vi "Create ipf File.vi"(2 "error in":errorcluster, 3 "Default ipf file path":path) -> (0 "error out":errorcluster, 1 "ipf file path":path)   [LabVIEW 2018]
doc: "This creats IPF file in selected location"
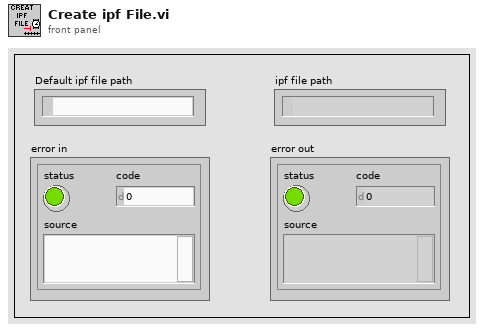
[diagram p1: front panel]
types:
  T1 = enum32{"invalid app kind", "Development System", "Run Time System", "Student Edition", "Embedded LabVIEW", "Evaluation", "Custom"}
  T2 = enum16{"open", "replace", "create", "open or create", "replace or create", "replace or create with confirmation"}
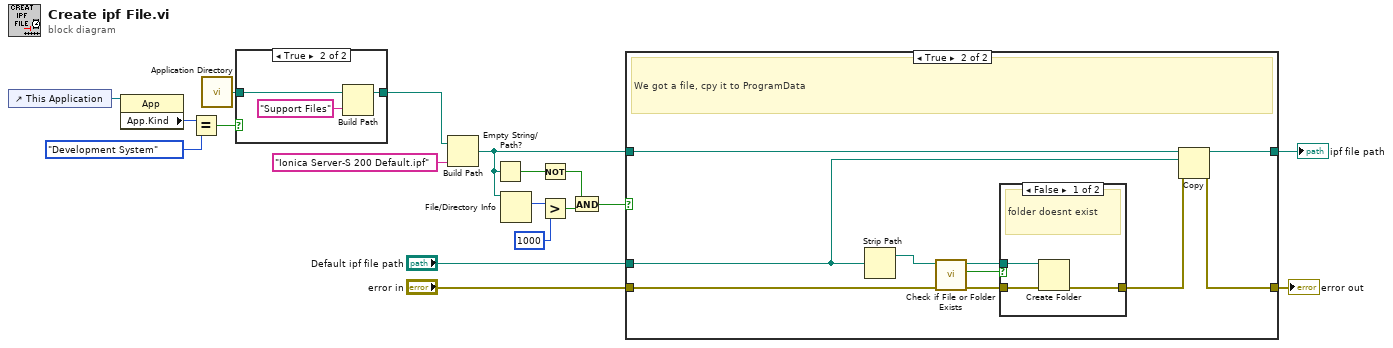
[diagram p0: block diagram]
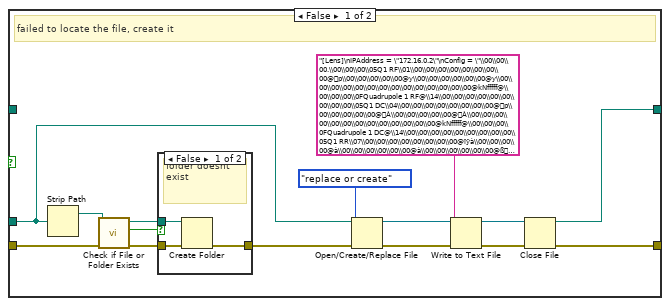
[diagram p3: hidden frame]
diagram:
  n1 = control-ref of="This Application"() -> (w6:refnum<vi>)
  n2 = property class="App"(reference=w6) -> ("App.Kind"=w5:T1)  [unwired: 1 in, 2 out]
  n3 = Equal?(x=w5, y=T1."Development System" ("Application:Kind")) -> (x = y?=w3:bool)
  n4 = call <vilib>:"Application Directory.vi"() -> ("Application Directory"=w2:path)
  n5 = case shown="True" w3 {
    tunnel: w2 -> [w19 w22]
    tunnel: [w19 w21] -> w1
    frame False {
    }
    frame True {
      n6 = Build Path(base path=w22, name or relative path="Support Files") -> (appended path=w21:path)
    }
  }
  n7 = Build Path(base path=w1, name or relative path="Ionica Server-S 200 Default.ipf") -> (appended path=w12:path)
  n8 = Empty String/Path?(string/path=w12) -> (empty?=w17:bool)
  n9 = File/Directory Info(path=w12) -> (size=w15:i64)  [unwired: 1 in, 6 out]
  n10 = Not(x=w17) -> (.not. x?=w16:bool)
  n11 = Greater?(x=w15, y=i64 1000) -> (0:w18:bool)
  n12 = And(x=w16, y=w18) -> (x .and. y?=w7:bool)
  n13 = case shown="True" w7 {
    tunnel: w12 -> [_ w51]
    tunnel: "error in" -> [w25 w47]
    tunnel: [w33 w50] -> w10
    tunnel: [w31 w49] -> w9
    tunnel: "Default ipf file path" -> [w24 w42]
    frame False {
      # "failed to locate the file, create it"
      n14 = Strip Path(path=w24) -> (stripped path=w28:path)  [unwired: 1 out]
      n15 = call <vilib>:"Check if File or Folder Exists.vi"("error in (no error)"=w25, "path"=w28) -> ("error out"=w30:errorcluster, "file or folder exists?"=w29:bool, "dup path"=w27:path)  [unwired: 7 in]
      n16 = case shown="False" w29 {
        tunnel: [w40 w41] -> w26
        tunnel: w30 -> [w39 w41]
        tunnel: w27 -> [w38 _]
        frame False {
          # "folder doesnt exist"
          n17 = Create Folder(path (use dialog)=w38, error in=w39) -> (error out=w40:errorcluster)  [unwired: 1 in, 2 out]
        }
        frame True {
        }
      }
      n18 = Open/Create/Replace File(file path (use dialog)=w24, error in=w26, operation (0:open)=T2."replace or create") -> (refnum out=w35:refnum<file>, error out=w36:errorcluster)  [unwired: 3 in, 1 out]
      n19 = Write to Text File(file (use dialog)=w35, text="[Lens]\nIPAddress = \"172.16.0.2\"\nConfig = \"\\00\\00\\00.\\00\\00\\00\\05Q1 RF\\01\\00\\00\\00\\00\\00\\00\\00\\00@p\\00\\00\\00\\00\\00@y\\00\\00\\00\\00\\00\\00@y\\00\\00\\00\\00\\00\\00\\00\\00\\00\\00\\00\\00\\00\\00@kNfffff@\\00\\00\\00\\0FQuadrupole 1 RF@\\14\\00\\00\\00\\00\\00\\00\\00\\00\\00\\05Q1 DC\\04\\00\\00\\00\\00\\00\\00\\00\\00@p\\00\\00\\00\\00\\00@À\\00\\00\\00\\00\\00@À\\00\\00\\00\\00\\00\\00\\00\\00\\00\\00\\00\\00\\00@kNfffff@\\00\\00\\00\\0FQuadrupole 1 DC@\\14\\00\\00\\00\\00\\00\\00\\00\\00\\00\\05Q1 RR\\07\\00\\00\\00\\00\\00\\00\\00\\00@ïÿà\\00\\00\\00\\00@à\\00\\00\\00\\00\\00\\00@à\\00\\00\\00\\00\\00\\00@ßÀ\\00\\00\\00\\00?ð\\00\\00\\00\\00\\00\\00@\\00\\00\\00\\0FQuadrupole 1 PW@\\14\\00\\00\\00\\00\\00\\00\\00\\00\\00\\05Q2 RF\\02\\00\\00\\00\\00\\00\\00\\00\\00@p\\00\\00\\00\\00\\00@y\\00\\00\\00\\00\\00\\00@y\\00\\00\\00\\00\\00\\00\\00\\00\\00\\00\\00\\00\\00\\00@kNfffff@\\00\\00\\00\\0FQuadrupole 2 RF@\\14\\00\\00\\00\\00\\00\\00\\00\\00\\00\\05Q2 DC\\05\\00\\00\\00\\00\\00\\00\\00\\00@p\\00\\00\\00\\00\\00@À\\00\\00\\00\\00\\00@À\\00\\00\\00\\00\\00\\00\\00\\00\\00\\00\\00\\00\\00@kNfffff@\\00\\00\\00\\0FQuadrupole 2 DC@\\14\\00\\00\\00\\00\\00\\00\\00\\00\\00\\05Q2 RR\t\\00\\00\\00\\00\\00\\00\\00\\00@ïÿà\\00\\00\\00\\00@à\\00\\00\\00\\00\\00\\00@à\\00\\00\\00\\00\\00\\00@ß¹À\\00\\00\\00\\00?ð\\00\\00\\00\\00\\00\\00@\\00\\00\\00\\0FQuadrupole 2 PW@\\14\\00\\00\\00\\00\\00\\00\\00\\00\\00\\05M1 RF\\03\\00\\00\\00\\00\\00\\00\\00\\00@@\\00\\00\\00\\00\\00@Y\\00\\00\\00\\00\\00\\00@Y\\00\\00\\00\\00\\00\\00\\00\\00\\00\\00\\00\\00\\00\\00@-ffffff\\06\\00\\00\\00\\0EMultipole 1 RF@\\14\\00\\00\\00\\00\\00\\00\\00\\00\\00\\02EV\\14Ài\\00\\00\\00\\00\\00\\00@i\\00\\00\\00\\00\\00\\00\\00\\00\\00\\00\\00\\00\\00\\00\\00\\00\\00\\00\\00\\00\\00\\00@à\\00\\00\\00\\00\\00\\00ÀPlÌÌÌÌÍ\\07\\00\\00\\00\\10Entrance Voltage@\\14\\00\\00\\00\\00\\00\\00\\00\\00\\00\\02ED\\15Ày\\00\\00\\00\\00\\00\\00@y\\00\\00\\00\\00\\00\\00\\00\\00\\00\\00\\00\\00\\00\\00\\00\\00\\00\\00\\00\\00\\00\\00@à\\00\\00\\00\\00\\00\\00À``\\00\\00\\00\\00\\00\\07\\00\\00\\00\\0ANot Used 1@\\14\\00\\00\\00\\00\\00\\00\\00\\00\\00\\02M1\\13Ày\\00\\00\\00\\00\\00\\00@y\\00\\00\\00\\00\\00\\00\\00\\00\\00\\00\\00\\00\\00\\00\\00\\00\\00\\00\\00\\00\\00\\00@à\\00\\00\\00\\00\\00\\00ÀPfffffg\\07\\00\\00\\00\\0BMultipole 1@\\14\\00\\00\\00\\00\\00\\00\\00\\00\\00\\02L1\\12Ày\\00\\00\\00\\00\\00\\00@y\\00\\00\\00\\00\\00\\00\\00\\00\\00\\00\\00\\00\\00\\00\\00\\00\\00\\00\\00\\00\\00\\00@ßþ\\00\\00\\00\\00\\00ÀPy\\07\\00\\00\\00\\10Multipole Lens 1@\\14\\00\\00\\00\\00\\00\\00\\00\\00\\00\\02M2\\16Ày\\00\\00\\00\\00\\00\\00@y\\00\\00\\00\\00\\00\\00\\00\\00\\00\\00\\00\\00\\00\\00\\00\\00\\00\\00\\00\\00\\00\\00@ß÷Êé\\13\\1AÀPjü-ÙÊ\\07\\00\\00\\00\\0BMultipole 2@\\14\\00\\00\\00\\00\\00\\00\\00\\00\\00\\02L2\\0BÀy\\00\\00\\00\\00\\00\\00@y\\00\\00\\00\\00\\00\\00\\00\\00\\00\\00\\00\\00\\00\\00\\00\\00\\00\\00\\00\\00\\00\\00@à\\00\\00\\00\\00\\00\\00ÀPzáG®\\14{\\07\\00\\00\\00\\10Multipole Lens 2@\\14\\00\\00\\00\\00\\00\\00\\00\\00\\00\\02PF\\0CÀy\\00\\00\\00\\00\\00\\00@y\\00\\00\\00\\00\\00\\00À0\\00\\00\\00\\00\\00\\00@0\\00\\00\\00\\00\\00\\00@à\\00\\00\\00\\00\\00\\01ÀPs33333\\07\\00\\00\\00\\0BPrefilter 1@\\14\\00\\00\\00\\00\\00\\00\\00\\00\\00\\02Q1\\06ÀbÀ\\00\\00\\00\\00\\00@bÀ\\00\\00\\00\\00\\00¿ð\\00\\00\\00\\00\\00\\00?ð\\00\\00\\00\\00\\00\\00@ßüÀ\\00\\00\\00\\00À`i\\0B\\00\\00\\00\\0CQuadrupole 1@\\14\\00\\00\\00\\00\\00\\00\\00\\00\\00\\05CC L1\\0DÀy\\00\\00\\00\\00\\00\\00@y\\00\\00\\00\\00\\00\\00\\00\\00\\00\\00\\00\\00\\00\\00\\00\\00\\00\\00\\00\\00\\00\\00@à\\00\\00\\00\\00\\00\\01ÀPs33333\\07\\00\\00\\00\\15Collision Cell Lens 1@\\14\\00\\00\\00\\00\\00\\00\\00\\00\\00\\05CC L2\\0EÀy\\00\\00\\00\\00\\00\\00@y\\00\\00\\00\\00\\00\\00ÀY\\00\\00\\00\\00\\00\\00@Y\\00\\00\\00\\00\\00\\00@à\\00\\00\\00\\00\\00\\01ÀPs33333\\07\\00\\00\\00\\15Collision Cell Lens 2@\\14\\00\\00\\00\\00\\00\\00\\00\\00\\00\\02CC\\17Ày\\00\\00\\00\\00\\00\\00@y\\00\\00\\00\\00\\00\\00ÀI\\00\\00\\00\\00\\00\\00@I\\00\\00\\00\\00\\00\\00@à\\04\\1B|S\\18ÀPmñLboÜ\\07\\00\\00\\00\\10Collision Energy@\\14\\00\\00\\00\\00\\00\\00\\00\\00\\00\\05CC AF\\0AÀy\\00\\00\\00\\00\\00\\00@y\\00\\00\\00\\00\\00\\00@I\\00\\00\\00\\00\\00\\00ÀI\\00\\00\\00\\00\\00\\00@à\\00\\00\\00\\00\\00\\01ÀPs33333\\07\\00\\00\\00\\0BAxial Field@\\14\\00\\00\\00\\00\\00\\00\\00\\00\\00\\05CC L3\\0FÀy\\00\\00\\00\\00\\00\\00@y\\00\\00\\00\\00\\00\\00ÀJ@\\00\\00\\00\\00\\00@J@\\00\\00\\00\\00\\00@ß÷Æ÷ýoÓÀPr\\10\\05 \\\\F\\07\\00\\00\\00\\15Collision Cell Lens 3@\\14\\00\\00\\00\\00\\00\\00\\00\\00\\00\\05CC L4\\10Ày\\00\\00\\00\\00\\00\\00@y\\00\\00\\00\\00\\00\\00ÀR \\00\\00\\00\\00\\00@R \\00\\00\\00\\00\\00@à\\00\\00\\00\\00\\00\\00ÀPlÌÌÌÌÍ\\07\\00\\00\\00\\15Collision Cell Lens 4@\\14\\00\\00\\00\\00\\00\\00\\00\\00\\00\\02Q2\\08ÀbÀ\\00\\00\\00\\00\\00@bÀ\\00\\00\\00\\00\\00ÀK\\00\\00\\00\\00\\00\\00@K\\00\\00\\00\\00\\00\\00@ßý\\00\\00\\00\\00\\00À`i\\0B\\00\\00\\00\\0CQuadrupole 2@\\14\\00\\00\\00\\00\\00\\00\\00\\00\\00\\02ID\\11Ày\\00\\00\\00\\00\\00\\00@y\\00\\00\\00\\00\\00\\00ÀY\\00\\00\\00\\00\\00\\00@Y\\00\\00\\00\\00\\00\\00@à\\00\\00\\00\\00\\00\\01ÀPs33333\\07\\00\\00\\00\\12Detector Deflector@\\14\\00\\00\\00\\00\\00\\00\\00\\00\\00\\04DISC @$\\00\\00\\00\\00\\00\\00@@\\00\\00\\00\\00\\00@4\\00\\00\\00\\00\\00\\00@4\\00\\00\\00\\00\\00\\00À\\14\\00\\00\\00\\00\\00\\00?ó®\\14záG®\\12\\00\\00\\00\\0DDiscriminator@$\\00\\00\\00\\00\\00\\00\\00\\00\\00\\02DV\"\\00\\00\\00\\00\\00\\00\\00\\00@«X\\00\\00\\00\\00\\00@¥\\18\\00\\00\\00\\00\\00@¥\\18\\00\\00\\00\\00\\00\\00\\00\\00\\00\\00\\00\\00\\00?Ú;HÂ\\05c´\\12\\00\\00\\00\\10Detector Voltage@$\\00\\00\\00\\00\\00\\00\\00\\00\\00\\08DET hornÈ\\00\\00\\00\\00\\00\\00\\00\\00@µ|\\00\\00\\00\\00\\00@µ|\\00\\00\\00\\00\\00@µ|\\00\\00\\00\\00\\00\\00\\00\\00\\00\\00\\00\\00\\00?Ú»)\\1EÏÇ0\\10\\00\\00\\00\\0DDetector Horn@$\\00\\00\\00\\00\\00\\00\\00\\00\\00\\06LS400A$\\00\\00\\00\\00\\00\\00\\00\\00@z@\\00\\00\\00\\00\\00@z@\\00\\00\\00\\00\\00@z@\\00\\00\\00\\00\\00\\00\\00\\00\\00\\00\\00\\00\\00@!\\04§Jy\\05@\\00\\00\\00\\18Lens Power Supply A +400@\\14\\00\\00\\00\\00\\00\\00\\00\\00\\00\\07LS-400A%Àz@\\00\\00\\00\\00\\00ÀT\\00\\00\\00\\00\\00\\00Àz@\\00\\00\\00\\00\\00Àz@\\00\\00\\00\\00\\00Àx%<SÆÀ!\\0Dö°ßk\\0E@\\00\\00\\00\\18Lens Power Supply A -400@\\14\\00\\00\\00\\00\\00\\00\\00\\00\\00\\06LS400B&\\00\\00\\00\\00\\00\\00\\00\\00@z@\\00\\00\\00\\00\\00@z@\\00\\00\\00\\00\\00@z@\\00\\00\\00\\00\\00\\00\\00\\00\\00\\00\\00\\00\\00@ ×Û%ö!@\\00\\00\\00\\18Lens Power Supply B +400@\\14\\00\\00\\00\\00\\00\\00\\00\\00\\00\\07LS-400B'Àz@\\00\\00\\00\\00\\00ÀT\\00\\00\\00\\00\\00\\00Àz@\\00\\00\\00\\00\\00Àz@\\00\\00\\00\\00\\00À´%\\03\\15$À ó©£xJ\\06@\\00\\00\\00\\19Lens Power Supply B  -400@\\14\\00\\00\\00\\00\\00\\00\\00\\00\\00\\06QPS800(\\00\\00\\00\\00\\00\\00\\00\\00@À\\00\\00\\00\\00\\00@À\\00\\00\\00\\00\\00@À\\00\\00\\00\\00\\00\\00\\00\\00\\00\\00\\00\\00\\00@\\11LÌÌÌÌÍ@\\00\\00\\00\\16Quad Power Supply +800@\\14\\00\\00\\00\\00\\00\\00\\00\\00\\00\\07QPS-800)ÀÀ\\00\\00\\00\\00\\00Àa\\00\\00\\00\\00\\00ÀÀ\\00\\00\\00\\00\\00ÀÀ\\00\\00\\00\\00\\00ÀÖ^ü^ýÀ\\11{ò\\19{ò\\1A@\\00\\00\\00\\16Quad Power Supply -800@\\14\\00\\00\\00\\00\\00\\00\\00\\00\\00\\02DG\\1A@D\\00\\00\\00\\00\\00\\00@rÀ\\00\\00\\00\\00\\00@T\\00\\00\\00\\00\\00\\00@T\\00\\00\\00\\00\\00\\00\\00\\00\\00\\00\\00\\00\\00\\00@@aë\\1E¸R \\00\\00\\00\\0ADrying Gas@@\\00\\00\\00\\00\\00\\00\\00\\00\\03NG1\\1B\\00\\00\\00\\00\\00\\00\\00\\00@@\\00\\00\\00\\00\\00\\00\\00\\00\\00\\00\\00\\00\\00\\00\\00\\00\\00\\00\\00\\00\\00\\00\\00\\00\\00\\00\\00\\00\\00@@aë\\1E¸R \\00\\00\\00\\0FNebulizer Gas 1@@\\00\\00\\00\\00\\00\\00\\00\\00\\03HG1\\1D\\00\\00\\00\\00\\00\\00\\00\\00@uà\\00\\00\\00\\00\\00\\00\\00\\00\\00\\00\\00\\00\\00\\00\\00\\00\\00\\00\\00\\00\\00\\00\\00\\00\\00\\00\\00\\00\\00@@aë\\1E¸R \\00\\00\\00\\0DHeating Gas 1@@\\00\\00\\00\\00\\00\\00\\00\\00\\03NG2\\1C\\00\\00\\00\\00\\00\\00\\00\\00@@\\00\\00\\00\\00\\00\\00\\00\\00\\00\\00\\00\\00\\00\\00\\00\\00\\00\\00\\00\\00\\00\\00\\00\\00\\00\\00\\00\\00\\00@@aë\\1E¸R \\00\\00\\00\\0FNebulizer Gas 2@@\\00\\00\\00\\00\\00\\00\\00\\00\\03HG2\\1E\\00\\00\\00\\00\\00\\00\\00\\00@uà\\00\\00\\00\\00\\00\\00\\00\\00\\00\\00\\00\\00\\00\\00\\00\\00\\00\\00\\00\\00\\00\\00\\00\\00\\00\\00\\00\\00\\00@@aë\\1E¸R \\00\\00\\00\\0DHeating Gas 2@@\\00\\00\\00\\00\\00\\00\\00\\00\\04CC P+\\00\\00\\00\\00\\00\\00\\00\\00@@\\00\\00\\00\\00\\00\\00\\00\\00\\00\\00\\00\\00\\00\\00\\00\\00\\00\\00\\00\\00\\00\\00\\00\\00\\00\\00\\00\\00\\00@@aë\\1E¸R\\06\\00\\00\\00\\12Collision Pressure@§p\\00\\00\\00\\00\\00\\00\\00\\00\\02SX*\\00\\00\\00\\00\\00\\00\\00\\00@@\\00\\00\\00\\00\\00\\00\\00\\00\\00\\00\\00\\00\\00\\00\\00\\00\\00\\00\\00\\00\\00\\00\\00\\00\\00\\00\\00\\00\\00@@aë\\1E¸R \\00\\00\\00\\0ESource Exhaust@@\\00\\00\\00\\00\\00\\00\\00\\00\\04ISV2ÌÀ¶Ú\\00\\00\\00\\00\\00@¶Ú\\00\\00\\00\\00\\00\\00\\00\\00\\00\\00\\00\\00\\00\\00\\00\\00\\00\\00\\00\\00\\00\\00\\00\\00\\00\\00\\00\\00\\00?¦R½<6\\114\"\\00\\00\\00\\0FElectroSpray V2@$\\00\\00\\00\\00\\00\\00\\00\\00\\00\\04ISV1ËÀ¶Ú\\00\\00\\00\\00\\00@¶Ú\\00\\00\\00\\00\\00\\00\\00\\00\\00\\00\\00\\00\\00\\00\\00\\00\\00\\00\\00\\00\\00\\00\\00\\00\\00\\00\\00\\00\\00?¦R½<6\\114\"\\00\\00\\00\\0FElectroSpray V1@$\\00\\00\\00\\00\\00\\00\\00\\00\\00\\02CDÊÀ\\14\\00\\00\\00\\00\\00\\00@\\14\\00\\00\\00\\00\\00\\00\\00\\00\\00\\00\\00\\00\\00\\00\\00\\00\\00\\00\\00\\00\\00\\00\\00\\00\\00\\00\\00\\00\\00\\00@I\\00\\00\\00\\00\\00\"\\00\\00\\00\\10Corona Discharge@$\\00\\00\\00\\00\\00\\00\\00\\00\\00\\03CAPÉÀ0\\00\\00\\00\\00\\00@0\\00\\00\\00\\00\\00\\00\\00\\00\\00\\00\\00\\00\\00\\00\\00\\00\\00\\00\\00\\00\\00\\00\\00\\00\\00\\00\\00\\00\\00?Ì(õÂ\\\\)\"\\00\\00\\00\\0BCurtain Cap@$\\00\\00\\00\\00\\00\\00\\00\\00\\00\\06HSID TQ\\00\\00\\00\\00\\00\\00\\00\\00@t\\00\\00\\00\\00\\00\\00@t\\00\\00\\00\\00\\00\\00@t\\00\\00\\00\\00\\00\\00\\00\\00\\00\\00\\00\\00\\00\\00?ð\\00\\00\\00\\00\\00\\00 \\00\\00\\00\\10HSID Temperature@§p\\00\\00\\00\\00\\00\\00\\00\\00\\04P1 TV\\00\\00\\00\\00\\00\\00\\00\\00@@\\00\\00\\00\\00\\00\\00\\00\\00\\00\\00\\00\\00\\00\\00\\00\\00\\00\\00\\00\\00\\00\\00\\00\\00\\00\\00\\00\\00\\00?ð\\00\\00\\00\\00\\00\\00 \\00\\00\\00\\0DSource 1 Temp@§p\\00\\00\\00\\00\\00\\00\\00\\00\\04P2 TT\\00\\00\\00\\00\\00\\00\\00\\00@@\\00\\00\\00\\00\\00\\00\\00\\00\\00\\00\\00\\00\\00\\00\\00\\00\\00\\00\\00\\00\\00\\00\\00\\00\\00\\00\\00\\00\\00?ð\\00\\00\\00\\00\\00\\00 \\00\\00\\00\\0DSource 2 Temp@§p\\00\\00\\00\\00\\00\\00\\00\\00\\10\\00\\00\\00WC:\\\\Users\\\\Public\\\\Simplicity 3Q\\\\3Q Service\\\\Current\\\\Config\\\\Config-S 200 Default-151217.c3n\\00\\00\\00\\0F210BC604140002P\\00\\00\\00\\0AQSight 210\\00\\00\\00\\0210\\00\\00\\00\\0220\\00\\00\\00\\043000\\00\\00\\00\\043000\\00\\00\\00\\0A172.16.0.2\\00\\00\\00\\01F\\00\\00\\00\\010\\00\\00\\00\\132864776525 47837346\\00\\00\\00\\132864776525 47837346\\00\\00\\00\\132864776499 66400194\\00\\00\\00\\013\\00\\00\\00\\011\\00\\00\\00\\011\"\nCal = \"\\00\\00\\00\\08\\00\\00\\00\\02@Mfffff@¿ø¥Å¤ð¯@]EÂ\\\\(ö@Ï£^U©9@eä(õÂ\\\\@×¨¶Ä\\19@x\\04ÌÌÌÌÍ@éö} AÆ@C®\\14záH@õQß\\10j@U\\\\(õÂ@ÿI\\0CR\\0F­z@¸Që\\1FA\\05\\0B8\\1AÙþ@<fffffA\t­\\0E*\"\nCal2 = \"\\00\\00\\00\\08\\00\\00\\00\\02@Mfffff@ÀVì±m¢0@]EÂ\\\\(ö@Ð+\\1DA@K@eä(õÂ\\\\@Ø0ïfOÛ¾@x\\04ÌÌÌÌÍ@çÍd¼ù@C®\\14záH@õ\\00-\\15þH,@U\\\\(õÂ@ÿ¹Ï\\12n@@¸Që\\1FA\\05÷]qÇ@<fffffA\tìú?®x\"\nCal3 = \"\\00\\00\\00\\08\\00\\00\\00\\02@F\\00\\00\\00\\00\\00@¸m¢Tã\\05î@`¢áG®\\14{@Ñlwi¡@o%p£×\\0A=@á!DÉ«GØ@}TÌÌÌÌÍ@ðiÀ5tÝ@@K\\1E¸Që@ô_Ò!\\10_¤@-\\1E¸QëA\\00H×¢.¡@\\1FfffffA\\05\\1Fâ&ÊÆÚ@À\\00\\00\\00\\00\\00A\t(/?ãá \"\nCal4 = \"\\00\\00\\00\\06\\00\\00\\00\\02@F\\00\\00\\00\\00\\00@¸[å\\19 c@K\\1E¸Që@ô/ð\\00\\00\\00\\00@-\\1E¸QëA\\00\\19@\\00\\00\\00\\00@\\1FfffffA\\05\\1A8\\00\\00\\00\\00@ï¸Që\\1FA\\07\\1A¸\\00\\00\\00\\00@À\\00\\00\\00\\00\\00A\t\\1B \\00\\00\\00\\00\"\nRes = \"\\00\\00\\00\\08\\00\\00\\00\\02@Mfffff@Ü@\\00\\00\\00\\00@]EÂ\\\\(ö@Ý\\15\\00\\00\\00\\00@eä(õÂ\\\\@Ýx@\\00\\00\\00\\00@x¼¸Që\\1F@Þð\\00\\00\\00\\00@C®\\14záH@à>à\\00\\00\\00\\00@U\\\\(õÂ@á2\\00\\00\\00\\00@¸Që\\1F@âLà\\00\\00\\00\\00@<fffff@ã\\11À\\00\\00\\00\\00\"\nRes2 = \"\\00\\00\\00\\06\\00\\00\\00\\02@Mfffff@Þ\\00\\00\\00\\00@eä(õÂ\\\\@Þo@\\00\\00\\00\\00@C®\\14záH@Ýj@\\00\\00\\00\\00@U\\\\(õÂ@Ü°@\\00\\00\\00\\00@¸Që\\1F@ÛÈ@\\00\\00\\00\\00@<fffff@Û+\\00\\00\\00\\00\\00\"\nRes3 = \"\\00\\00\\00\\08\\00\\00\\00\\02@Mfffff@ß@ÿþ°@]EÂ\\\\(ö@ß·¬\\00\\14u@eä(õÂ\\\\@à\\13ß#Ý\\15@x\\04ÌÌÌÌÍ@à·Í¸þ\\1F@C®\\14záH@áw\\0EìE@U\\\\(õÂ@áI\\00 \\00\\00\\00@¸Që\\1F@â^a@\\00\\00\\00@<fffff@ã\\1CÁ#ÔÌ\"\nRes4 = \"\\00\\00\\00\\08\\00\\00\\00\\02@Mfffff@Þµ>\\13=°~@]EÂ\\\\(ö@Þ~1Cfíà@eä(õÂ\\\\@Þ5¦²Ar\\00@x\\04ÌÌÌÌÍ@Þ%¥\\1C¸äB@C®\\14záH@Û»fhß@U\\\\(õÂ@Úý°ÈØÆÁ@¸Që\\1F@Ú\\17\\15KK\\08=@<fffff@Ùçb\\07¶Ð\"\nRes5 = \"\\00\\00\\00\\08\\00\\00\\00\\02@Mfffff@Ü@\\00\\00\\00\\00@]EÂ\\\\(ö@Ý\\15\\00\\00\\00\\00@eä(õÂ\\\\@Ýx@\\00\\00\\00\\00@x¼¸Që\\1F@Þð\\00\\00\\00\\00@C®\\14záH@à>à\\00\\00\\00\\00@U\\\\(õÂ@á2\\00\\00\\00\\00@¸Që\\1F@âLà\\00\\00\\00\\00@<fffff@ã\\11À\\00\\00\\00\\00\"\nRes6 = \"\\00\\00\\00\\06\\00\\00\\00\\02@Mfffff@Þ\\00\\00\\00\\00@eä(õÂ\\\\@Þo@\\00\\00\\00\\00@C®\\14záH@Ýj@\\00\\00\\00\\00@U\\\\(õÂ@Ü°@\\00\\00\\00\\00@¸Që\\1F@ÛÈ@\\00\\00\\00\\00@<fffff@Û+\\00\\00\\00\\00\\00\"\nRes7 = \"\\00\\00\\00\\06\\00\\00\\00\\02@F\\00\\00\\00\\00\\00@ÞêÀ\\00\\00\\00\\00@K\\1E¸Që@ÛÚ\\00\\00\\00\\00\\00@-\\1E¸Që@ÙéÀ\\00\\00\\00\\00@\\1Ffffff@Ø+\\00\\00\\00\\00@ï¸Që\\1F@×w\\00\\00\\00\\00@À\\00\\00\\00\\00\\00@ÖË@\\00\\00\\00\\00\"\nRes8 = \"\\00\\00\\00\\06\\00\\00\\00\\02@F\\00\\00\\00\\00\\00@ß£À\\00\\00\\00\\00@K\\1E¸Që@Þ~@\\00\\00\\00\\00@-\\1E¸Që@ÝÀ\\00\\00\\00\\00@\\1Ffffff@ÜÆ\\00\\00\\00\\00@ï¸Që\\1F@Ü_À\\00\\00\\00\\00@À\\00\\00\\00\\00\\00@Ü\\12\\00\\00\\00\\00\"\nRes9 = \"\\00\\00\\00\\08\\00\\00\\00\\02@F\\00\\00\\00\\00\\00@à\\11luGa©@`¢áG®\\14{@à \\1D©z@o%p£×\\0A=@Þ¶%\\15{×@}TÌÌÌÌÍ@Ý\\08×1#î½@K\\1E¸Që@ÜQÿ`\\00\\00\\00@-\\1E¸Që@Ù¶P\\03Ì¨@\\1Ffffff@×ùônÈE@À\\00\\00\\00\\00\\00@ÖÀ< 3s\\0A\"\nRes10 = \"\\00\\00\\00\\06\\00\\00\\00\\02@F\\00\\00\\00\\00\\00@àgþiy±È@K\\1E¸Që@â\\1DÀ\\00\\00\\00\\00@-\\1E¸Që@ã'À\\00\\00\\00\\00@\\1Ffffff@ä\\05\\00\\00\\00\\00\\00@ï¸Që\\1F@äbÀ\\00\\00\\00\\00@À\\00\\00\\00\\00\\00@äÀ\\00\\00\\00\\00\"\nRes11 = \"\\00\\00\\00\\06\\00\\00\\00\\02@F\\00\\00\\00\\00\\00@ÞÀ\\00\\00\\00\\00@K\\1E¸Që@Û¨\\00\\00\\00\\00\\00@-\\1E¸Që@ÙÀ\\00\\00\\00\\00@\\1Ffffff@×Ç\\00\\00\\00\\00@ï¸Që\\1F@×\\13\\00\\00\\00\\00@À\\00\\00\\00\\00\\00@Ög@\\00\\00\\00\\00\"\nRes12 = \"\\00\\00\\00\\06\\00\\00\\00\\02@F\\00\\00\\00\\00\\00@ß?À\\00\\00\\00\\00@K\\1E¸Që@Þ\\1A@\\00\\00\\00\\00@-\\1E¸Që@Ý2À\\00\\00\\00\\00@\\1Ffffff@Üb\\00\\00\\00\\00@ï¸Që\\1F@ÛûÀ\\00\\00\\00\\00@À\\00\\00\\00\\00\\00@Û®\\00\\00\\00\\00\"\nConfigFile = \"/C/Users/Public/Simplicity 3Q/3Q Service/Current/Config/Config-S 200 Default-151217.c3n\"\nDeadTime = 0\nUseDT = FALSE\nTableFiles = \"\\00\\00\\00\\10PTH0\\00\\00\\00X\\00\\00\\00\\06\\01U\\15Default Startup Files\\0AAll Tables\\12Pending-Series 200\\07Cal-Res\\15Q1 Pos-P20-130905.calPTH0\\00\\00\\00X\\00\\00\\00\\06\\01U\\15Default Startup Files\\0AAll Tables\\12Pending-Series 200\\07Cal-Res\\15Q2 Pos-P20-130905.calPTH0\\00\\00\\00X\\00\\00\\00\\06\\01U\\15Default Startup Files\\0AAll Tables\\12Pending-Series 200\\07Cal-Res\\15Q1 Neg-P20-130905.calPTH0\\00\\00\\00X\\00\\00\\00\\06\\01U\\15Default Startup Files\\0AAll Tables\\12Pending-Series 200\\07Cal-Res\\15Q2 Neg-P20-130905.calPTH0\\00\\00\\00<\\00\\00\\00\\06\\01C\\05Users\\03Lab\\07Desktop\\0DServerTesting\\15My Resolution bad.resPTH0\\00\\00\\00T\\00\\00\\00\\06\\01U\\15Default Startup Files\\0AAll Tables\\12Pending-Series 200\\07Cal-Res\\11Q2 Pos-130905.resPTH0\\00\\00\\008\\00\\00\\00\\06\\01C\\05Users\\03Lab\\07Desktop\\0DServerTesting\\11My Resolution.resPTH0\\00\\00\\00T\\00\\00\\00\\06\\01U\\15Default Startup Files\\0AAll Tables\\12Pending-Series 200\\07Cal-Res\\11Q2 Pos-130905.resPTH0\\00\\00\\00<\\00\\00\\00\\06\\01C\\05Users\\03Lab\\07Desktop\\0DServerTesting\\15My Resolution bad.resPTH0\\00\\00\\00T\\00\\00\\00\\06\\01U\\15Default Startup Files\\0AAll Tables\\12Pending-Series 200\\07Cal-Res\\11Q2 Pos-130905.resPTH0\\00\\00\\00T\\00\\00\\00\\06\\01U\\15Default Startup Files\\0AAll Tables\\12Pending-Series 200\\07Cal-Res\\11Q1 Neg-130905.resPTH0\\00\\00\\00T\\00\\00\\00\\06\\01U\\15Default Startup Files\\0AAll Tables\\12Pending-Series 200\\07Cal-Res\\11Q2 Neg-130905.resPTH0\\00\\00\\00T\\00\\00\\00\\06\\01U\\15Default Startup Files\\0AAll Tables\\12Pending-Series 200\\07Cal-Res\\11Q1 Neg-130905.resPTH0\\00\\00\\00T\\00\\00\\00\\06\\01U\\15Default Startup Files\\0AAll Tables\\12Pending-Series 200\\07Cal-Res\\11Q2 Neg-130905.resPTH0\\00\\00\\00T\\00\\00\\00\\06\\01U\\15Default Startup Files\\0AAll Tables\\12Pending-Series 200\\07Cal-Res\\11Q1 Neg-130905.resPTH0\\00\\00\\00T\\00\\00\\00\\06\\01U\\15Default Startup Files\\0AAll Tables\\12Pending-Series 200\\07Cal-Res\\11Q2 Neg-130905.res\"\nTuneFile = \"\"\nScanParam = FALSE\nCtrWid = FALSE\nScanR = \"\\00\\00\\00\\00\\00\\00\\00\\00\\00\\00\\00\\00\\00@Y\\00\\00\\00\\00\\00\\00?ð\\00\\00\\00\\00\\00\\00\\00\"\nPolOp = FALSE\nDiagFile = \"\"\nCCLogics = 0\nCILogics = 0\nShowServer = True\nLog path = \"/C/ProgramData/PerkinElmer/Simplicity/Logs\"\nUpsIP = \"\"\nSimplicity Server Log File Name = \"Simplicity.Server.log\"\nIonSniffer Log File Name = \"Ion.Sniffer.log\"\nService Tools Log File Name = \"Service.Tools.log\"\nLCType = 0\n\n[ADC]\nRow0-Col0 = \"0\"\nRow0-Col1 = \"DET HORN, V\"\nRow0-Col2 = \"0\"\nRow0-Col3 = \"181.818182\"\nRow0-Col4 = \"41890.909091\"\nRow0-Col5 = \"0\"\nRow0-Col6 = \"250.000\"\nRow0-Col7 = \"0.000\"\nRow1-Col0 = \"1\"\nRow1-Col1 = \"DET BIAS, V\"\nRow1-Col2 = \"0\"\nRow1-Col3 = \"100.000000\"\nRow1-Col4 = \"40960.000000\"\nRow1-Col5 = \"0\"\nRow1-Col6 = \"250.000\"\nRow1-Col7 = \"0.000\"\nRow2-Col0 = \"2\"\nRow2-Col1 = \"Discriminator\"\nRow2-Col2 = \"0\"\nRow2-Col3 = \"-0.727273\"\nRow2-Col4 = \"1042.618182\"\nRow2-Col5 = \"0\"\nRow2-Col6 = \"5.000\"\nRow2-Col7 = \"0.000\"\nRow3-Col0 = \"3\"\nRow3-Col1 = \"HED, V\"\nRow3-Col2 = \"0\"\nRow3-Col3 = \"0.000000\"\nRow3-Col4 = \"2013.866667\"\nRow3-Col5 = \"0\"\nRow3-Col6 = \"250.000\"\nRow3-Col7 = \"0.000\"\nRow4-Col0 = \"4\"\nRow4-Col1 = \"DET Spare5\"\nRow4-Col2 = \"0\"\nRow4-Col3 = \"0.000000\"\nRow4-Col4 = \"1.000000\"\nRow4-Col5 = \"0\"\nRow4-Col6 = \"0.000\"\nRow4-Col7 = \"0.000\"\nRow5-Col0 = \"5\"\nRow5-Col1 = \"DET Spare6\"\nRow5-Col2 = \"0\"\nRow5-Col3 = \"0.000000\"\nRow5-Col4 = \"1.000000\"\nRow5-Col5 = \"0\"\nRow5-Col6 = \"0.000\"\nRow5-Col7 = \"0.000\"\nRow6-Col0 = \"6\"\nRow6-Col1 = \"DET Spare7\"\nRow6-Col2 = \"0\"\nRow6-Col3 = \"0.000000\"\nRow6-Col4 = \"1.000000\"\nRow6-Col5 = \"0\"\nRow6-Col6 = \"0.000\"\nRow6-Col7 = \"0.000\"\nRow7-Col0 = \"7\"\nRow7-Col1 = \"DET Spare8\"\nRow7-Col2 = \"0\"\nRow7-Col3 = \"0.000000\"\nRow7-Col4 = \"1.000000\"\nRow7-Col5 = \"0\"\nRow7-Col6 = \"0.000\"\nRow7-Col7 = \"0.000\"\nRow8-Col0 = \"8\"\nRow8-Col1 = \"Main SystemCUR (A)\"\nRow8-Col2 = \"0\"\nRow8-Col3 = \"0.000000\"\nRow8-Col4 = \"3.000000\"\nRow8-Col5 = \"0\"\nRow8-Col6 = \"0.000\"\nRow8-Col7 = \"0.000\"\nRow9-Col0 = \"9\"\nRow9-Col1 = \"AC Box Spare\"\nRow9-Col2 = \"0\"\nRow9-Col3 = \"0.000000\"\nRow9-Col4 = \"1.000000\"\nRow9-Col5 = \"0\"\nRow9-Col6 = \"0.000\"\nRow9-Col7 = \"0.000\"\nRow10-Col0 = \"10\"\nRow10-Col1 = \"+15V PS CUR (A)\"\nRow10-Col2 = \"0\"\nRow10-Col3 = \"-13.500000\"\nRow10-Col4 = \"5.400000\"\nRow10-Col5 = \"0\"\nRow10-Col6 = \"0.000\"\nRow10-Col7 = \"0.000\"\nRow11-Col0 = \"11\"\nRow11-Col1 = \"-15V PS CUR (A)\"\nRow11-Col2 = \"0\"\nRow11-Col3 = \"-13.500000\"\nRow11-Col4 = \"5.400000\"\nRow11-Col5 = \"0\"\nRow11-Col6 = \"0.000\"\nRow11-Col7 = \"0.000\"\nRow12-Col0 = \"12\"\nRow12-Col1 = \"+28V PS CUR (A)\"\nRow12-Col2 = \"0\"\nRow12-Col3 = \"-25.000000\"\nRow12-Col4 = \"10.000000\"\nRow12-Col5 = \"0\"\nRow12-Col6 = \"0.000\"\nRow12-Col7 = \"0.000\"\nRow13-Col0 = \"13\"\nRow13-Col1 = \"-28V PS CUR (A)\"\nRow13-Col2 = \"0\"\nRow13-Col3 = \"-25.000000\"\nRow13-Col4 = \"10.000000\"\nRow13-Col5 = \"0\"\nRow13-Col6 = \"0.000\"\nRow13-Col7 = \"0.000\"\nRow14-Col0 = \"14\"\nRow14-Col1 = \"+58V PS CUR (A)\"\nRow14-Col2 = \"0\"\nRow14-Col3 = \"-25.000000\"\nRow14-Col4 = \"10.000000\"\nRow14-Col5 = \"0\"\nRow14-Col6 = \"0.000\"\nRow14-Col7 = \"0.000\"\nRow15-Col0 = \"15\"\nRow15-Col1 = \"+24V PS CUR (A)\"\nRow15-Col2 = \"0\"\nRow15-Col3 = \"-25.000000\"\nRow15-Col4 = \"10.000000\"\nRow15-Col5 = \"0\"\nRow15-Col6 = \"0.000\"\nRow15-Col7 = \"0.000\"\nRow16-Col0 = \"16\"\nRow16-Col1 = \"Q1 DC POLE A, V\"\nRow16-Col2 = \"0\"\nRow16-Col3 = \"0.490196\"\nRow16-Col4 = \"200.784314\"\nRow16-Col5 = \"0\"\nRow16-Col6 = \"5.000\"\nRow16-Col7 = \"0.000\"\nRow17-Col0 = \"17\"\nRow17-Col1 = \"Q1 DC POLE B, V\"\nRow17-Col2 = \"0\"\nRow17-Col3 = \"0.487805\"\nRow17-Col4 = \"199.804878\"\nRow17-Col5 = \"0\"\nRow17-Col6 = \"5.000\"\nRow17-Col7 = \"0.000\"\nRow18-Col0 = \"18\"\nRow18-Col1 = \"Q2 DC POLE A, V\"\nRow18-Col2 = \"0\"\nRow18-Col3 = \"0.492611\"\nRow18-Col4 = \"201.773399\"\nRow18-Col5 = \"0\"\nRow18-Col6 = \"5.000\"\nRow18-Col7 = \"0.000\"\nRow19-Col0 = \"19\"\nRow19-Col1 = \"Q2 DC POLE B, V\"\nRow19-Col2 = \"0\"\nRow19-Col3 = \"0.487805\"\nRow19-Col4 = \"199.804878\"\nRow19-Col5 = \"0\"\nRow19-Col6 = \"5.000\"\nRow19-Col7 = \"0.000\"\nRow20-Col0 = \"20\"\nRow20-Col1 = \"Quad DC PS +600 V\"\nRow20-Col2 = \"0\"\nRow20-Col3 = \"0.128866\"\nRow20-Col4 = \"200.577320\"\nRow20-Col5 = \"0\"\nRow20-Col6 = \"10.000\"\nRow20-Col7 = \"0.000\"\nRow21-Col0 = \"21\"\nRow21-Col1 = \"Quad DC PS -600 V\"\nRow21-Col2 = \"0\"\nRow21-Col3 = \"-2.686567\"\nRow21-Col4 = \"200.869936\"\nRow21-Col5 = \"0\"\nRow21-Col6 = \"10.000\"\nRow21-Col7 = \"0.000\"\nRow22-Col0 = \"22\"\nRow22-Col1 = \"QDC PS +CUR (A)\"\nRow22-Col2 = \"0\"\nRow22-Col3 = \"0.000000\"\nRow22-Col4 = \"0.004600\"\nRow22-Col5 = \"0\"\nRow22-Col6 = \"0.000\"\nRow22-Col7 = \"0.000\"\nRow23-Col0 = \"23\"\nRow23-Col1 = \"QDC PS -CUR (A)\"\nRow23-Col2 = \"0\"\nRow23-Col3 = \"0.000000\"\nRow23-Col4 = \"0.004600\"\nRow23-Col5 = \"0\"\nRow23-Col6 = \"0.000\"\nRow23-Col7 = \"0.000\"\nRow24-Col0 = \"24\"\nRow24-Col1 = \"Q2 RF Pk-Pk, V\"\nRow24-Col2 = \"0\"\nRow24-Col3 = \"0.000000\"\nRow24-Col4 = \"-1208.000000\"\nRow24-Col5 = \"0\"\nRow24-Col6 = \"0.000\"\nRow24-Col7 = \"0.000\"\nRow25-Col0 = \"25\"\nRow25-Col1 = \"Q2 RF HS1 TEMP, C\"\nRow25-Col2 = \"0\"\nRow25-Col3 = \"0.000000\"\nRow25-Col4 = \"100.000000\"\nRow25-Col5 = \"0\"\nRow25-Col6 = \"0.000\"\nRow25-Col7 = \"0.000\"\nRow26-Col0 = \"26\"\nRow26-Col1 = \"Q2 RF HS2 TEMP, C\"\nRow26-Col2 = \"0\"\nRow26-Col3 = \"0.000000\"\nRow26-Col4 = \"100.000000\"\nRow26-Col5 = \"0\"\nRow26-Col6 = \"0.000\"\nRow26-Col7 = \"0.000\"\nRow27-Col0 = \"27\"\nRow27-Col1 = \"Q2 TUNING DC, V\"\nRow27-Col2 = \"0\"\nRow27-Col3 = \"0.000000\"\nRow27-Col4 = \"3.000000\"\nRow27-Col5 = \"0\"\nRow27-Col6 = \"0.200\"\nRow27-Col7 = \"0.000\"\nRow28-Col0 = \"28\"\nRow28-Col1 = \"Q2 RF Spare5\"\nRow28-Col2 = \"0\"\nRow28-Col3 = \"0.000000\"\nRow28-Col4 = \"1.000000\"\nRow28-Col5 = \"0\"\nRow28-Col6 = \"0.000\"\nRow28-Col7 = \"0.000\"\nRow29-Col0 = \"29\"\nRow29-Col1 = \"Q2 RF Spare6\"\nRow29-Col2 = \"0\"\nRow29-Col3 = \"0.000000\"\nRow29-Col4 = \"1.000000\"\nRow29-Col5 = \"0\"\nRow29-Col6 = \"0.000\"\nRow29-Col7 = \"0.000\"\nRow30-Col0 = \"30\"\nRow30-Col1 = \"Q2 RF Spare7\"\nRow30-Col2 = \"0\"\nRow30-Col3 = \"0.000000\"\nRow30-Col4 = \"1.000000\"\nRow30-Col5 = \"0\"\nRow30-Col6 = \"0.000\"\nRow30-Col7 = \"0.000\"\nRow31-Col0 = \"31\"\nRow31-Col1 = \"Q2 RF Spare8\"\nRow31-Col2 = \"0\"\nRow31-Col3 = \"0.000000\"\nRow31-Col4 = \"1.000000\"\nRow31-Col5 = \"0\"\nRow31-Col6 = \"0.000\"\nRow31-Col7 = \"0.000\"\nRow32-Col0 = \"32\"\nRow32-Col1 = \"CC AF +/-400, V\"\nRow32-Col2 = \"0\"\nRow32-Col3 = \"0.370943\"\nRow32-Col4 = \"101.292117\"\nRow32-Col5 = \"0\"\nRow32-Col6 = \"10.000\"\nRow32-Col7 = \"0.000\"\nRow33-Col0 = \"33\"\nRow33-Col1 = \"L2 +/-400, V\"\nRow33-Col2 = \"0\"\nRow33-Col3 = \"0.000000\"\nRow33-Col4 = \"101.386139\"\nRow33-Col5 = \"0\"\nRow33-Col6 = \"5.000\"\nRow33-Col7 = \"0.000\"\nRow34-Col0 = \"34\"\nRow34-Col1 = \"PF +/-400, V\"\nRow34-Col2 = \"0\"\nRow34-Col3 = \"0.124611\"\nRow34-Col4 = \"102.080997\"\nRow34-Col5 = \"0\"\nRow34-Col6 = \"10.000\"\nRow34-Col7 = \"0.000\"\nRow35-Col0 = \"35\"\nRow35-Col1 = \"CC L1 +/-400, V\"\nRow35-Col2 = \"0\"\nRow35-Col3 = \"0.123724\"\nRow35-Col4 = \"101.354779\"\nRow35-Col5 = \"0\"\nRow35-Col6 = \"10.000\"\nRow35-Col7 = \"0.000\"\nRow36-Col0 = \"36\"\nRow36-Col1 = \"CC L2 +/-400, V\"\nRow36-Col2 = \"0\"\nRow36-Col3 = \"0.000000\"\nRow36-Col4 = \"101.011097\"\nRow36-Col5 = \"0\"\nRow36-Col6 = \"10.000\"\nRow36-Col7 = \"0.000\"\nRow37-Col0 = \"37\"\nRow37-Col1 = \"CC L3 +/-400, V\"\nRow37-Col2 = \"0\"\nRow37-Col3 = \"-0.247678\"\nRow37-Col4 = \"101.448916\"\nRow37-Col5 = \"0\"\nRow37-Col6 = \"10.000\"\nRow37-Col7 = \"0.000\"\nRow38-Col0 = \"38\"\nRow38-Col1 = \"CC L4 +/-400, V\"\nRow38-Col2 = \"0\"\nRow38-Col3 = \"0.249532\"\nRow38-Col4 = \"102.208359\"\nRow38-Col5 = \"0\"\nRow38-Col6 = \"10.000\"\nRow38-Col7 = \"0.000\"\nRow39-Col0 = \"39\"\nRow39-Col1 = \"ID +/-400, V\"\nRow39-Col2 = \"0\"\nRow39-Col3 = \"0.123877\"\nRow39-Col4 = \"101.480334\"\nRow39-Col5 = \"0\"\nRow39-Col6 = \"10.000\"\nRow39-Col7 = \"0.000\"\nRow40-Col0 = \"40\"\nRow40-Col1 = \"L1 +/-400, V\"\nRow40-Col2 = \"0\"\nRow40-Col3 = \"0.246914\"\nRow40-Col4 = \"101.135802\"\nRow40-Col5 = \"0\"\nRow40-Col6 = \"5.000\"\nRow40-Col7 = \"0.000\"\nRow41-Col0 = \"41\"\nRow41-Col1 = \"M1 +/-400, V\"\nRow41-Col2 = \"0\"\nRow41-Col3 = \"0.124224\"\nRow41-Col4 = \"101.763975\"\nRow41-Col5 = \"0\"\nRow41-Col6 = \"5.000\"\nRow41-Col7 = \"0.000\"\nRow42-Col0 = \"42\"\nRow42-Col1 = \"EV +/-400, V\"\nRow42-Col2 = \"0\"\nRow42-Col3 = \"0.248447\"\nRow42-Col4 = \"101.763975\"\nRow42-Col5 = \"0\"\nRow42-Col6 = \"6.000\"\nRow42-Col7 = \"0.000\"\nRow43-Col0 = \"43\"\nRow43-Col1 = \"Spare +/-400, V\"\nRow43-Col2 = \"0\"\nRow43-Col3 = \"1.000000\"\nRow43-Col4 = \"100.000000\"\nRow43-Col5 = \"0\"\nRow43-Col6 = \"5.000\"\nRow43-Col7 = \"0.000\"\nRow44-Col0 = \"44\"\nRow44-Col1 = \"M2 +/-400, V\"\nRow44-Col2 = \"0\"\nRow44-Col3 = \"-0.123916\"\nRow44-Col4 = \"101.511772\"\nRow44-Col5 = \"0\"\nRow44-Col6 = \"5.000\"\nRow44-Col7 = \"0.000\"\nRow45-Col0 = \"45\"\nRow45-Col1 = \"CC +/-400, V\"\nRow45-Col2 = \"0\"\nRow45-Col3 = \"0.496278\"\nRow45-Col4 = \"101.637717\"\nRow45-Col5 = \"0\"\nRow45-Col6 = \"5.000\"\nRow45-Col7 = \"0.000\"\nRow46-Col0 = \"46\"\nRow46-Col1 = \"Spare +/-400, V\"\nRow46-Col2 = \"0\"\nRow46-Col3 = \"0.000000\"\nRow46-Col4 = \"100.000000\"\nRow46-Col5 = \"0\"\nRow46-Col6 = \"0.000\"\nRow46-Col7 = \"0.000\"\nRow47-Col0 = \"47\"\nRow47-Col1 = \"Spare +/-400, V\"\nRow47-Col2 = \"0\"\nRow47-Col3 = \"-1.500000\"\nRow47-Col4 = \"100.000000\"\nRow47-Col5 = \"0\"\nRow47-Col6 = \"0.000\"\nRow47-Col7 = \"0.000\"\nRow48-Col0 = \"48\"\nRow48-Col1 = \"Q1 RF Pk-Pk, V\"\nRow48-Col2 = \"0\"\nRow48-Col3 = \"0.000000\"\nRow48-Col4 = \"-1221.000000\"\nRow48-Col5 = \"0\"\nRow48-Col6 = \"0.000\"\nRow48-Col7 = \"0.000\"\nRow49-Col0 = \"49\"\nRow49-Col1 = \"Q1 RF HS1 TEMP, C\"\nRow49-Col2 = \"0\"\nRow49-Col3 = \"0.000000\"\nRow49-Col4 = \"100.000000\"\nRow49-Col5 = \"0\"\nRow49-Col6 = \"0.000\"\nRow49-Col7 = \"0.000\"\nRow50-Col0 = \"50\"\nRow50-Col1 = \"Q1 RF HS2 TEMP, C\"\nRow50-Col2 = \"0\"\nRow50-Col3 = \"0.000000\"\nRow50-Col4 = \"100.000000\"\nRow50-Col5 = \"0\"\nRow50-Col6 = \"0.000\"\nRow50-Col7 = \"0.000\"\nRow51-Col0 = \"51\"\nRow51-Col1 = \"Q1 TUNING DC, V\"\nRow51-Col2 = \"0\"\nRow51-Col3 = \"0.000000\"\nRow51-Col4 = \"3.000000\"\nRow51-Col5 = \"0\"\nRow51-Col6 = \"0.200\"\nRow51-Col7 = \"0.000\"\nRow52-Col0 = \"52\"\nRow52-Col1 = \"Q1 RF Spare5\"\nRow52-Col2 = \"0\"\nRow52-Col3 = \"0.000000\"\nRow52-Col4 = \"1.000000\"\nRow52-Col5 = \"0\"\nRow52-Col6 = \"0.000\"\nRow52-Col7 = \"0.000\"\nRow53-Col0 = \"53\"\nRow53-Col1 = \"Q1 RF Spare6\"\nRow53-Col2 = \"0\"\nRow53-Col3 = \"0.000000\"\nRow53-Col4 = \"1.000000\"\nRow53-Col5 = \"0\"\nRow53-Col6 = \"0.000\"\nRow53-Col7 = \"0.000\"\nRow54-Col0 = \"54\"\nRow54-Col1 = \"Q1 RF Spare7\"\nRow54-Col2 = \"0\"\nRow54-Col3 = \"0.000000\"\nRow54-Col4 = \"1.000000\"\nRow54-Col5 = \"0\"\nRow54-Col6 = \"0.000\"\nRow54-Col7 = \"0.000\"\nRow55-Col0 = \"55\"\nRow55-Col1 = \"Q1 RF Spare8\"\nRow55-Col2 = \"0\"\nRow55-Col3 = \"0.000000\"\nRow55-Col4 = \"1.000000\"\nRow55-Col5 = \"0\"\nRow55-Col6 = \"0.000\"\nRow55-Col7 = \"0.000\"\nRow56-Col0 = \"56\"\nRow56-Col1 = \"M1 RF Pk-Pk, V\"\nRow56-Col2 = \"0\"\nRow56-Col3 = \"0.000000\"\nRow56-Col4 = \"-885.000000\"\nRow56-Col5 = \"0\"\nRow56-Col6 = \"15.000\"\nRow56-Col7 = \"0.000\"\nRow57-Col0 = \"57\"\nRow57-Col1 = \"M1 RF HS1 TEMP, C\"\nRow57-Col2 = \"0\"\nRow57-Col3 = \"0.000000\"\nRow57-Col4 = \"100.000000\"\nRow57-Col5 = \"0\"\nRow57-Col6 = \"0.000\"\nRow57-Col7 = \"0.000\"\nRow58-Col0 = \"58\"\nRow58-Col1 = \"M1 RF HS2 TEMP, C\"\nRow58-Col2 = \"0\"\nRow58-Col3 = \"0.000000\"\nRow58-Col4 = \"100.000000\"\nRow58-Col5 = \"0\"\nRow58-Col6 = \"0.000\"\nRow58-Col7 = \"0.000\"\nRow59-Col0 = \"59\"\nRow59-Col1 = \"M1 TUNING DC, V\"\nRow59-Col2 = \"0\"\nRow59-Col3 = \"0.000000\"\nRow59-Col4 = \"3.000000\"\nRow59-Col5 = \"0\"\nRow59-Col6 = \"0.200\"\nRow59-Col7 = \"0.000\"\nRow60-Col0 = \"60\"\nRow60-Col1 = \"M1 RF Spare5\"\nRow60-Col2 = \"0\"\nRow60-Col3 = \"0.000000\"\nRow60-Col4 = \"1.000000\"\nRow60-Col5 = \"0\"\nRow60-Col6 = \"0.000\"\nRow60-Col7 = \"0.000\"\nRow61-Col0 = \"61\"\nRow61-Col1 = \"M1 RF Spare6\"\nRow61-Col2 = \"0\"\nRow61-Col3 = \"0.000000\"\nRow61-Col4 = \"1.000000\"\nRow61-Col5 = \"0\"\nRow61-Col6 = \"0.000\"\nRow61-Col7 = \"0.000\"\nRow62-Col0 = \"62\"\nRow62-Col1 = \"M1 RF Spare7\"\nRow62-Col2 = \"0\"\nRow62-Col3 = \"0.000000\"\nRow62-Col4 = \"1.000000\"\nRow62-Col5 = \"0\"\nRow62-Col6 = \"0.000\"\nRow62-Col7 = \"0.000\"\nRow63-Col0 = \"63\"\nRow63-Col1 = \"M1 RF Spare8\"\nRow63-Col2 = \"0\"\nRow63-Col3 = \"0.000000\"\nRow63-Col4 = \"1.000000\"\nRow63-Col5 = \"0\"\nRow63-Col6 = \"0.000\"\nRow63-Col7 = \"0.000\"\nRow64-Col0 = \"64\"\nRow64-Col1 = \"Drying Gas Output, V\"\nRow64-Col2 = \"0\"\nRow64-Col3 = \"-14.830000\"\nRow64-Col4 = \"107.610001\"\nRow64-Col5 = \"0\"\nRow64-Col6 = \"15.000\"\nRow64-Col7 = \"0.000\"\nRow65-Col0 = \"65\"\nRow65-Col1 = \"Neb Gas 1 Out, V\"\nRow65-Col2 = \"0\"\nRow65-Col3 = \"-14.830000\"\nRow65-Col4 = \"107.610001\"\nRow65-Col5 = \"0\"\nRow65-Col6 = \"25.000\"\nRow65-Col7 = \"0.000\"\nRow66-Col0 = \"66\"\nRow66-Col1 = \"Neb Gas 2 Out, V\"\nRow66-Col2 = \"0\"\nRow66-Col3 = \"-14.830000\"\nRow66-Col4 = \"107.610001\"\nRow66-Col5 = \"0\"\nRow66-Col6 = \"25.000\"\nRow66-Col7 = \"0.000\"\nRow67-Col0 = \"67\"\nRow67-Col1 = \"Heater Gas 1 Out, V\"\nRow67-Col2 = \"0\"\nRow67-Col3 = \"-14.830000\"\nRow67-Col4 = \"107.610001\"\nRow67-Col5 = \"0\"\nRow67-Col6 = \"40.000\"\nRow67-Col7 = \"0.000\"\nRow68-Col0 = \"68\"\nRow68-Col1 = \"Heater Gas 2 Out, V\"\nRow68-Col2 = \"0\"\nRow68-Col3 = \"-14.830000\"\nRow68-Col4 = \"107.610001\"\nRow68-Col5 = \"0\"\nRow68-Col6 = \"40.000\"\nRow68-Col7 = \"0.000\"\nRow69-Col0 = \"69\"\nRow69-Col1 = \"Gas box Spare6\"\nRow69-Col2 = \"0\"\nRow69-Col3 = \"0.000000\"\nRow69-Col4 = \"1.000000\"\nRow69-Col5 = \"0\"\nRow69-Col6 = \"0.000\"\nRow69-Col7 = \"0.000\"\nRow70-Col0 = \"70\"\nRow70-Col1 = \"SourceExhaust on/off\"\nRow70-Col2 = \"0\"\nRow70-Col3 = \"0.000000\"\nRow70-Col4 = \"1.000000\"\nRow70-Col5 = \"0\"\nRow70-Col6 = \"0.000\"\nRow70-Col7 = \"0.000\"\nRow71-Col0 = \"71\"\nRow71-Col1 = \"CC Gas 0-18 V, V\"\nRow71-Col2 = \"0\"\nRow71-Col3 = \"0.000000\"\nRow71-Col4 = \"100.000000\"\nRow71-Col5 = \"0\"\nRow71-Col6 = \"2.000\"\nRow71-Col7 = \"0.000\"\nRow72-Col0 = \"72\"\nRow72-Col1 = \"S Exhaust reading\"\nRow72-Col2 = \"0\"\nRow72-Col3 = \"0.000000\"\nRow72-Col4 = \"36.000000\"\nRow72-Col5 = \"0\"\nRow72-Col6 = \"0.000\"\nRow72-Col7 = \"0.000\"\nRow73-Col0 = \"73\"\nRow73-Col1 = \"Press Spare2\"\nRow73-Col2 = \"0\"\nRow73-Col3 = \"0.000000\"\nRow73-Col4 = \"1.000000\"\nRow73-Col5 = \"0\"\nRow73-Col6 = \"0.000\"\nRow73-Col7 = \"0.000\"\nRow74-Col0 = \"74\"\nRow74-Col1 = \"Foreline Press, torr\"\nRow74-Col2 = \"0\"\nRow74-Col3 = \"1.850000\"\nRow74-Col4 = \"4.500000\"\nRow74-Col5 = \"0\"\nRow74-Col6 = \"0.000\"\nRow74-Col7 = \"0.000\"\nRow75-Col0 = \"75\"\nRow75-Col1 = \"Press Spare4\"\nRow75-Col2 = \"0\"\nRow75-Col3 = \"0.000000\"\nRow75-Col4 = \"1.000000\"\nRow75-Col5 = \"0\"\nRow75-Col6 = \"0.000\"\nRow75-Col7 = \"0.000\"\nRow76-Col0 = \"76\"\nRow76-Col1 = \"Drying Gas Input P (V)\"\nRow76-Col2 = \"0\"\nRow76-Col3 = \"-40.898998\"\nRow76-Col4 = \"29.875000\"\nRow76-Col5 = \"0\"\nRow76-Col6 = \"20.000\"\nRow76-Col7 = \"0.000\"\nRow77-Col0 = \"77\"\nRow77-Col1 = \"Press Spare6\"\nRow77-Col2 = \"0\"\nRow77-Col3 = \"0.000000\"\nRow77-Col4 = \"1.000000\"\nRow77-Col5 = \"0\"\nRow77-Col6 = \"0.000\"\nRow77-Col7 = \"0.000\"\nRow78-Col0 = \"78\"\nRow78-Col1 = \"Gas Manifold Input P (V)\"\nRow78-Col2 = \"0\"\nRow78-Col3 = \"-40.898998\"\nRow78-Col4 = \"29.875000\"\nRow78-Col5 = \"0\"\nRow78-Col6 = \"20.000\"\nRow78-Col7 = \"0.000\"\nRow79-Col0 = \"79\"\nRow79-Col1 = \"Press Spare8\"\nRow79-Col2 = \"0\"\nRow79-Col3 = \"0.000000\"\nRow79-Col4 = \"1.000000\"\nRow79-Col5 = \"0\"\nRow79-Col6 = \"0.000\"\nRow79-Col7 = \"0.000\"\nRow80-Col0 = \"80\"\nRow80-Col1 = \"AC Box Spare\"\nRow80-Col2 = \"0\"\nRow80-Col3 = \"0.000000\"\nRow80-Col4 = \"1.000000\"\nRow80-Col5 = \"0\"\nRow80-Col6 = \"0.000\"\nRow80-Col7 = \"0.000\"\nRow81-Col0 = \"81\"\nRow81-Col1 = \"28V (+)\"\nRow81-Col2 = \"0\"\nRow81-Col3 = \"0.000000\"\nRow81-Col4 = \"5.800000\"\nRow81-Col5 = \"0\"\nRow81-Col6 = \"1.000\"\nRow81-Col7 = \"0.000\"\nRow82-Col0 = \"82\"\nRow82-Col1 = \"28V (-)\"\nRow82-Col2 = \"0\"\nRow82-Col3 = \"0.000000\"\nRow82-Col4 = \"5.800000\"\nRow82-Col5 = \"0\"\nRow82-Col6 = \"1.000\"\nRow82-Col7 = \"0.000\"\nRow83-Col0 = \"83\"\nRow83-Col1 = \"58V (+)\"\nRow83-Col2 = \"0\"\nRow83-Col3 = \"0.000000\"\nRow83-Col4 = \"12.000000\"\nRow83-Col5 = \"0\"\nRow83-Col6 = \"15.000\"\nRow83-Col7 = \"0.000\"\nRow84-Col0 = \"84\"\nRow84-Col1 = \"AC Box Spare\"\nRow84-Col2 = \"0\"\nRow84-Col3 = \"0.000000\"\nRow84-Col4 = \"1.000000\"\nRow84-Col5 = \"0\"\nRow84-Col6 = \"0.000\"\nRow84-Col7 = \"0.000\"\nRow85-Col0 = \"85\"\nRow85-Col1 = \"24V (+)\"\nRow85-Col2 = \"0\"\nRow85-Col3 = \"0.000000\"\nRow85-Col4 = \"5.110000\"\nRow85-Col5 = \"0\"\nRow85-Col6 = \"1.000\"\nRow85-Col7 = \"0.000\"\nRow86-Col0 = \"86\"\nRow86-Col1 = \"15V (+)\"\nRow86-Col2 = \"0\"\nRow86-Col3 = \"0.000000\"\nRow86-Col4 = \"3.180000\"\nRow86-Col5 = \"0\"\nRow86-Col6 = \"1.000\"\nRow86-Col7 = \"0.000\"\nRow87-Col0 = \"87\"\nRow87-Col1 = \"15V (-)\"\nRow87-Col2 = \"0\"\nRow87-Col3 = \"0.000000\"\nRow87-Col4 = \"3.180000\"\nRow87-Col5 = \"0\"\nRow87-Col6 = \"1.000\"\nRow87-Col7 = \"0.000\"\nRow88-Col0 = \"88\"\nRow88-Col1 = \"LN2 PS Pos (V)\"\nRow88-Col2 = \"0\"\nRow88-Col3 = \"0.113065\"\nRow88-Col4 = \"100.341709\"\nRow88-Col5 = \"0\"\nRow88-Col6 = \"20.000\"\nRow88-Col7 = \"0.000\"\nRow89-Col0 = \"89\"\nRow89-Col1 = \"LN2 PS Neg (V)\"\nRow89-Col2 = \"0\"\nRow89-Col3 = \"-1.557678\"\nRow89-Col4 = \"100.819985\"\nRow89-Col5 = \"0\"\nRow89-Col6 = \"20.000\"\nRow89-Col7 = \"0.000\"\nRow90-Col0 = \"90\"\nRow90-Col1 = \"LN2 PS +CUR (A)\"\nRow90-Col2 = \"0\"\nRow90-Col3 = \"0.000000\"\nRow90-Col4 = \"0.004600\"\nRow90-Col5 = \"0\"\nRow90-Col6 = \"0.000\"\nRow90-Col7 = \"0.000\"\nRow91-Col0 = \"91\"\nRow91-Col1 = \"LN2 PS -CUR (A)\"\nRow91-Col2 = \"0\"\nRow91-Col3 = \"0.000000\"\nRow91-Col4 = \"0.004600\"\nRow91-Col5 = \"0\"\nRow91-Col6 = \"0.000\"\nRow91-Col7 = \"0.000\"\nRow92-Col0 = \"92\"\nRow92-Col1 = \"Lens Board 2 +5V\"\nRow92-Col2 = \"0\"\nRow92-Col3 = \"0.000000\"\nRow92-Col4 = \"1.000000\"\nRow92-Col5 = \"0\"\nRow92-Col6 = \"0.200\"\nRow92-Col7 = \"0.000\"\nRow93-Col0 = \"93\"\nRow93-Col1 = \"Lens Board 2 -5V\"\nRow93-Col2 = \"0\"\nRow93-Col3 = \"0.000000\"\nRow93-Col4 = \"1.000000\"\nRow93-Col5 = \"0\"\nRow93-Col6 = \"0.200\"\nRow93-Col7 = \"0.000\"\nRow94-Col0 = \"94\"\nRow94-Col1 = \"LN2 HVPS Reference\"\nRow94-Col2 = \"0\"\nRow94-Col3 = \"0.000000\"\nRow94-Col4 = \"1.000000\"\nRow94-Col5 = \"0\"\nRow94-Col6 = \"0.200\"\nRow94-Col7 = \"0.000\"\nRow95-Col0 = \"95\"\nRow95-Col1 = \"L1-ADC12-8\"\nRow95-Col2 = \"0\"\nRow95-Col3 = \"0.000000\"\nRow95-Col4 = \"1.000000\"\nRow95-Col5 = \"0\"\nRow95-Col6 = \"0.000\"\nRow95-Col7 = \"0.000\"\nRow96-Col0 = \"96\"\nRow96-Col1 = \"LN1 PS Pos (V)\"\nRow96-Col2 = \"0\"\nRow96-Col3 = \"0.376648\"\nRow96-Col4 = \"100.278719\"\nRow96-Col5 = \"0\"\nRow96-Col6 = \"20.000\"\nRow96-Col7 = \"0.000\"\nRow97-Col0 = \"97\"\nRow97-Col1 = \"LN1 PS Neg (V)\"\nRow97-Col2 = \"0\"\nRow97-Col3 = \"-1.986804\"\nRow97-Col4 = \"100.598240\"\nRow97-Col5 = \"0\"\nRow97-Col6 = \"20.000\"\nRow97-Col7 = \"0.000\"\nRow98-Col0 = \"98\"\nRow98-Col1 = \"LN1 PS +CUR (A)\"\nRow98-Col2 = \"0\"\nRow98-Col3 = \"0.000000\"\nRow98-Col4 = \"0.017650\"\nRow98-Col5 = \"0\"\nRow98-Col6 = \"0.000\"\nRow98-Col7 = \"0.000\"\nRow99-Col0 = \"99\"\nRow99-Col1 = \"LN1 PS -CUR (A)\"\nRow99-Col2 = \"0\"\nRow99-Col3 = \"0.000000\"\nRow99-Col4 = \"0.017650\"\nRow99-Col5 = \"0\"\nRow99-Col6 = \"0.000\"\nRow99-Col7 = \"0.000\"\nRow100-Col0 = \"100\"\nRow100-Col1 = \"Lens Board 1 +5V\"\nRow100-Col2 = \"0\"\nRow100-Col3 = \"0.000000\"\nRow100-Col4 = \"1.000000\"\nRow100-Col5 = \"0\"\nRow100-Col6 = \"0.200\"\nRow100-Col7 = \"0.000\"\nRow101-Col0 = \"101\"\nRow101-Col1 = \"Lens Board 1 -5V\"\nRow101-Col2 = \"0\"\nRow101-Col3 = \"0.000000\"\nRow101-Col4 = \"1.000000\"\nRow101-Col5 = \"0\"\nRow101-Col6 = \"0.200\"\nRow101-Col7 = \"0.000\"\nRow102-Col0 = \"102\"\nRow102-Col1 = \"LN1 HVPS Reference\"\nRow102-Col2 = \"0\"\nRow102-Col3 = \"0.000000\"\nRow102-Col4 = \"1.000000\"\nRow102-Col5 = \"0\"\nRow102-Col6 = \"0.200\"\nRow102-Col7 = \"0.000\"\nRow103-Col0 = \"103\"\nRow103-Col1 = \"L3-ADC13-8\"\nRow103-Col2 = \"0\"\nRow103-Col3 = \"0.000000\"\nRow103-Col4 = \"1.000000\"\nRow103-Col5 = \"0\"\nRow103-Col6 = \"0.000\"\nRow103-Col7 = \"0.000\"\nRow104-Col0 = \"104\"\nRow104-Col1 = \"CAP Voltage\"\nRow104-Col2 = \"0\"\nRow104-Col3 = \"0.000000\"\nRow104-Col4 = \"13.900000\"\nRow104-Col5 = \"0\"\nRow104-Col6 = \"150.000\"\nRow104-Col7 = \"0.000\"\nRow105-Col0 = \"105\"\nRow105-Col1 = \"HSID T\"\nRow105-Col2 = \"0\"\nRow105-Col3 = \"0.000000\"\nRow105-Col4 = \"1.000000\"\nRow105-Col5 = \"0\"\nRow105-Col6 = \"30.000\"\nRow105-Col7 = \"0.000\"\nRow106-Col0 = \"106\"\nRow106-Col1 = \"CD Corona\"\nRow106-Col2 = \"0\"\nRow106-Col3 = \"0.000000\"\nRow106-Col4 = \"0.025000\"\nRow106-Col5 = \"0\"\nRow106-Col6 = \"0.400\"\nRow106-Col7 = \"0.000\"\nRow107-Col0 = \"107\"\nRow107-Col1 = \"ISV1 Voltage\"\nRow107-Col2 = \"0\"\nRow107-Col3 = \"0.000000\"\nRow107-Col4 = \"22.500000\"\nRow107-Col5 = \"0\"\nRow107-Col6 = \"350.000\"\nRow107-Col7 = \"0.000\"\nRow108-Col0 = \"108\"\nRow108-Col1 = \"Probe2 Temp\"\nRow108-Col2 = \"0\"\nRow108-Col3 = \"0.000000\"\nRow108-Col4 = \"1.000000\"\nRow108-Col5 = \"0\"\nRow108-Col6 = \"40.000\"\nRow108-Col7 = \"0.000\"\nRow109-Col0 = \"109\"\nRow109-Col1 = \"ISV2 Voltage\"\nRow109-Col2 = \"0\"\nRow109-Col3 = \"0.000000\"\nRow109-Col4 = \"24.000000\"\nRow109-Col5 = \"0\"\nRow109-Col6 = \"350.000\"\nRow109-Col7 = \"0.000\"\nRow110-Col0 = \"110\"\nRow110-Col1 = \"Probe1 Temp\"\nRow110-Col2 = \"0\"\nRow110-Col3 = \"0.000000\"\nRow110-Col4 = \"1.000000\"\nRow110-Col5 = \"0\"\nRow110-Col6 = \"40.000\"\nRow110-Col7 = \"0.000\"\nRow111-Col0 = \"111\"\nRow111-Col1 = \"PIC 87\"\nRow111-Col2 = \"0\"\nRow111-Col3 = \"0.000000\"\nRow111-Col4 = \"1.000000\"\nRow111-Col5 = \"0\"\nRow111-Col6 = \"0.000\"\nRow111-Col7 = \"0.000\"\nRow112-Col0 = \"112\"\nRow112-Col1 = \"PIC 88\"\nRow112-Col2 = \"0\"\nRow112-Col3 = \"0.000000\"\nRow112-Col4 = \"1.000000\"\nRow112-Col5 = \"0\"\nRow112-Col6 = \"0.000\"\nRow112-Col7 = \"0.000\"\nRow113-Col0 = \"113\"\nRow113-Col1 = \"PROBE 1 ID\"\nRow113-Col2 = \"0\"\nRow113-Col3 = \"0.000000\"\nRow113-Col4 = \"1.000000\"\nRow113-Col5 = \"0\"\nRow113-Col6 = \"0.000\"\nRow113-Col7 = \"0.000\"\nRow114-Col0 = \"114\"\nRow114-Col1 = \"PROBE 2 ID\"\nRow114-Col2 = \"0\"\nRow114-Col3 = \"0.000000\"\nRow114-Col4 = \"1.000000\"\nRow114-Col5 = \"0\"\nRow114-Col6 = \"0.000\"\nRow114-Col7 = \"0.000\"\nRow115-Col0 = \"115\"\nRow115-Col1 = \"PIC Spare\"\nRow115-Col2 = \"0\"\nRow115-Col3 = \"0.000000\"\nRow115-Col4 = \"1.000000\"\nRow115-Col5 = \"0\"\nRow115-Col6 = \"0.000\"\nRow115-Col7 = \"0.000\"\nRow116-Col0 = \"116\"\nRow116-Col1 = \"PIC Spare\"\nRow116-Col2 = \"0\"\nRow116-Col3 = \"0.000000\"\nRow116-Col4 = \"1.000000\"\nRow116-Col5 = \"0\"\nRow116-Col6 = \"0.000\"\nRow116-Col7 = \"0.000\"\nRow117-Col0 = \"117\"\nRow117-Col1 = \"PIC Spare\"\nRow117-Col2 = \"0\"\nRow117-Col3 = \"0.000000\"\nRow117-Col4 = \"1.000000\"\nRow117-Col5 = \"0\"\nRow117-Col6 = \"0.000\"\nRow117-Col7 = \"0.000\"\nRow118-Col0 = \"118\"\nRow118-Col1 = \"PIC Spare\"\nRow118-Col2 = \"0\"\nRow118-Col3 = \"0.000000\"\nRow118-Col4 = \"1.000000\"\nRow118-Col5 = \"0\"\nRow118-Col6 = \"0.000\"\nRow118-Col7 = \"0.000\"\nRow119-Col0 = \"119\"\nRow119-Col1 = \"VAC Gauge\"\nRow119-Col2 = \"0\"\nRow119-Col3 = \"0.000000\"\nRow119-Col4 = \"1.000000\"\nRow119-Col5 = \"0\"\nRow119-Col6 = \"0.000\"\nRow119-Col7 = \"0.000\"\nRow120-Col0 = \"120\"\nRow120-Col1 = \"Door Interlock\"\nRow120-Col2 = \"0\"\nRow120-Col3 = \"0.000000\"\nRow120-Col4 = \"1.000000\"\nRow120-Col5 = \"0\"\nRow120-Col6 = \"0.000\"\nRow120-Col7 = \"0.000\"\nRow121-Col0 = \"121\"\nRow121-Col1 = \"Vacuum Ready\"\nRow121-Col2 = \"0\"\nRow121-Col3 = \"0.000000\"\nRow121-Col4 = \"1.000000\"\nRow121-Col5 = \"0\"\nRow121-Col6 = \"0.000\"\nRow121-Col7 = \"0.000\"\nRow122-Col0 = \"122\"\nRow122-Col1 = \"LC1 Out1 Hold\"\nRow122-Col2 = \"0\"\nRow122-Col3 = \"0.000000\"\nRow122-Col4 = \"1.000000\"\nRow122-Col5 = \"0\"\nRow122-Col6 = \"0.000\"\nRow122-Col7 = \"0.000\"\nRow123-Col0 = \"123\"\nRow123-Col1 = \"LC1 Out2 Stop\"\nRow123-Col2 = \"0\"\nRow123-Col3 = \"0.000000\"\nRow123-Col4 = \"1.000000\"\nRow123-Col5 = \"0\"\nRow123-Col6 = \"0.000\"\nRow123-Col7 = \"0.000\"\nRow124-Col0 = \"124\"\nRow124-Col1 = \"LC2 Out1 Hold\"\nRow124-Col2 = \"0\"\nRow124-Col3 = \"0.000000\"\nRow124-Col4 = \"1.000000\"\nRow124-Col5 = \"0\"\nRow124-Col6 = \"0.000\"\nRow124-Col7 = \"0.000\"\nRow125-Col0 = \"125\"\nRow125-Col1 = \"LC2 Out2 Stop\"\nRow125-Col2 = \"0\"\nRow125-Col3 = \"0.000000\"\nRow125-Col4 = \"1.000000\"\nRow125-Col5 = \"0\"\nRow125-Col6 = \"0.000\"\nRow125-Col7 = \"0.000\"\nRow126-Col0 = \"126\"\nRow126-Col1 = \"LC1 In\"\nRow126-Col2 = \"0\"\nRow126-Col3 = \"0.000000\"\nRow126-Col4 = \"1.000000\"\nRow126-Col5 = \"0\"\nRow126-Col6 = \"0.000\"\nRow126-Col7 = \"0.000\"\nRow127-Col0 = \"127\"\nRow127-Col1 = \"LC2 In\"\nRow127-Col2 = \"0\"\nRow127-Col3 = \"0.000000\"\nRow127-Col4 = \"1.000000\"\nRow127-Col5 = \"0\"\nRow127-Col6 = \"0.000\"\nRow127-Col7 = \"0.000\"\nRow# = 0\n\n[Window]\nMain = \"\\00Í\\00W\\036\\00Ï\"\nTuning = \"\\02(\\00\\02\\05\\01\\02N\"\nServer = \"\\01&\\00¾\\04z\\02?\"\nDiagnostic2 = \\01\\14\\00h\\03í\\02\n\n[PIC]\nCEMPol = FALSE\n\n[Oscillator0]\nRefClk = \"10\"\nClkMult = \"10\"\nFreqOut = \"1.4950\"\nScaleF = \"0.4\"\n\n[Oscillator]\n0 = \\00\\00\\00\\03ªÁ\\05µ\\02Öwp\\00\\00\\00\\00\n1 = \\00\\00\\00\\03ªÁ\\05µ\\02Öwp\\00\\00\\00\\01\n2 = \\00\\00\\00\\03ªÁ\\05µ\\03âÖ$\\00\\00\\00\\02\nChip = 2\n\n[Oscillator1]\nRefClk = \"10\"\nClkMult = \"10\"\nFreqOut = \"1.1151\"\nScaleF = \"0.6\"\n\n[Oscillator2]\nRefClk = \"10\"\nClkMult = \"10\"\nFreqOut = \"1.1151\"\nScaleF = \"0.6\"\n\n[AutoCal]\nMethodFolder = \"/C/Users/Public/Instrument/AutoCal/MS Methods\"\nReferenceFolder = \"/C/Users/Public/Instrument/Configuration/Current setting/Calibration\"\nParameterFolder = \"/C/ProgramData/PerkinElmer/Simplicity\"\nReportFolder = \"/C/Users/Public/Instrument/AutoCal\"\nLastPositive = \"08/04/2017 09:14:42\"\nPositiveQ1Result = \"\\00\\00\\00\\08\\00\\00\\00\\0A\\00\\00\\00\\0559.05\\00\\00\\00\\0559.09\\00\\00\\00\\040.04\\00\\00\\00\\040.74\\00\\00\\00\\078.12E+6\\00\\00\\00\\078288.90\\00\\00\\00\\06138.61\\00\\00\\00\\0833081.45\\00\\00\\00\\048.62\\00\\00\\00\\06Passed\\00\\00\\00\\06117.09\\00\\00\\00\\06117.10\\00\\00\\00\\040.01\\00\\00\\00\\040.71\\00\\00\\00\\072.21E+7\\00\\00\\00\\0816333.58\\00\\00\\00\\06138.61\\00\\00\\00\\0833582.00\\00\\00\\00\\048.62\\00\\00\\00\\06Passed\\00\\00\\00\\06175.13\\00\\00\\00\\06175.11\\00\\00\\00\\05-0.02\\00\\00\\00\\040.80\\00\\00\\00\\073.32E+7\\00\\00\\00\\0824376.39\\00\\00\\00\\06138.57\\00\\00\\00\\0833977.46\\00\\00\\00\\046.81\\00\\00\\00\\06Passed\\00\\00\\00\\06384.30\\00\\00\\00\\06384.27\\00\\00\\00\\05-0.03\\00\\00\\00\\040.76\\00\\00\\00\\073.10E+7\\00\\00\\00\\0853403.54\\00\\00\\00\\06138.77\\00\\00\\00\\0835483.01\\00\\00\\00\\047.20\\00\\00\\00\\06Passed\\00\\00\\00\\06616.46\\00\\00\\00\\06616.47\\00\\00\\00\\040.01\\00\\00\\00\\040.78\\00\\00\\00\\071.02E+7\\00\\00\\00\\0885621.07\\00\\00\\00\\06138.77\\00\\00\\00\\0837071.49\\00\\00\\00\\046.93\\00\\00\\00\\06Passed\\00\\00\\00\\06906.67\\00\\00\\00\\06906.71\\00\\00\\00\\040.04\\00\\00\\00\\040.77\\00\\00\\00\\071.29E+6\\00\\00\\00\t125904.62\\00\\00\\00\\06138.81\\00\\00\\00\\0839020.07\\00\\00\\00\\046.71\\00\\00\\00\\06Passed\\00\\00\\00\\071254.93\\00\\00\\00\\071254.99\\00\\00\\00\\040.06\\00\\00\\00\\040.79\\00\\00\\00\\077.07E+4\\00\\00\\00\t174266.18\\00\\00\\00\\06138.87\\00\\00\\00\\0841279.03\\00\\00\\00\\046.49\\00\\00\\00\\06Passed\\00\\00\\00\\071487.10\\00\\00\\00\\071487.09\\00\\00\\00\\05-0.01\\00\\00\\00\\040.71\\00\\00\\00\\072.20E+4\\00\\00\\00\t206517.95\\00\\00\\00\\06138.91\\00\\00\\00\\0842854.31\\00\\00\\00\\046.79\\00\\00\\00\\06Passed\"\nLastNegative = \"08/02/2017 12:58:56\"\nNegativeQ1Result = \"\\00\\00\\00\\08\\00\\00\\00\\0A\\00\\00\\00\\0545.00\\00\\00\\00\\0545.02\\00\\00\\00\\040.02\\00\\00\\00\\040.77\\00\\00\\00\\072.78E+7\\00\\00\\00\\076341.66\\00\\00\\00\\06138.73\\00\\00\\00\\0832936.33\\00\\00\\00\\047.78\\00\\00\\00\\06Passed\\00\\00\\00\\06133.09\\00\\00\\00\\06133.12\\00\\00\\00\\040.03\\00\\00\\00\\040.80\\00\\00\\00\\071.39E+5\\00\\00\\00\\0818543.34\\00\\00\\00\\06138.51\\00\\00\\00\\0833653.01\\00\\00\\00\\048.14\\00\\00\\00\\06Passed\\00\\00\\00\\06249.17\\00\\00\\00\\06249.21\\00\\00\\00\\040.04\\00\\00\\00\\040.79\\00\\00\\00\\077.11E+4\\00\\00\\00\\0834640.14\\00\\00\\00\\06138.81\\00\\00\\00\\0834500.13\\00\\00\\00\\047.83\\00\\00\\00\\06Passed\\00\\00\\00\\06469.30\\00\\00\\00\\06469.22\\00\\00\\00\\05-0.08\\00\\00\\00\\040.79\\00\\00\\00\\071.47E+6\\00\\00\\00\\0865203.24\\00\\00\\00\\06138.84\\00\\00\\00\\0836030.71\\00\\00\\00\\046.95\\00\\00\\00\\06Passed\\00\\00\\00\\06585.39\\00\\00\\00\\06585.39\\00\\00\\00\\05-0.00\\00\\00\\00\\040.74\\00\\00\\00\\071.64E+6\\00\\00\\00\\0881307.98\\00\\00\\00\\06138.73\\00\\00\\00\\0836839.50\\00\\00\\00\\047.27\\00\\00\\00\\06Passed\\00\\00\\00\\06933.64\\00\\00\\00\\06933.59\\00\\00\\00\\05-0.05\\00\\00\\00\\040.66\\00\\00\\00\\072.84E+6\\00\\00\\00\t129660.61\\00\\00\\00\\06138.84\\00\\00\\00\\0839200.00\\00\\00\\00\\046.78\\00\\00\\00\\06Passed\\00\\00\\00\\071223.85\\00\\00\\00\\071223.84\\00\\00\\00\\05-0.01\\00\\00\\00\\040.68\\00\\00\\00\\073.15E+5\\00\\00\\00\t169951.06\\00\\00\\00\\06138.83\\00\\00\\00\\0841118.36\\00\\00\\00\\046.61\\00\\00\\00\\06Passed\\00\\00\\00\\071456.00\\00\\00\\00\\071455.97\\00\\00\\00\\05-0.03\\00\\00\\00\\040.65\\00\\00\\00\\072.59E+4\\00\\00\\00\t202192.81\\00\\00\\00\\06138.88\\00\\00\\00\\0842674.10\\00\\00\\00\\046.70\\00\\00\\00\\06Passed\"\n\n[Report]\nRefMass = \\00\\00\\00\\08@``\\00\\00\\00\\00\\00@eÀ\\00\\00\\00\\00\\00@h`\\00\\00\\00\\00\\00@xÐ\\00\\00\\00\\00\\00@|\\00\\00\\00\\00\\00\\00@\\0Afffff@\\12fffff@\\1Afffff\nLensList = \"\\00\\00\\00\\1B\\00\\00\\00\\03\\00\\00\\00\\14\\00\\00\\00\\13\\00\\00\\00\\12\\00\\00\\00\\16\\00\\00\\00\\0B\\00\\00\\00\\0C\\00\\00\\00\\06\\00\\00\\00\\0D\\00\\00\\00\\0E\\00\\00\\00\\17\\00\\00\\00\\0A\\00\\00\\00\\0F\\00\\00\\00\\10\\00\\00\\00\\08\\00\\00\\00\\11\\00\\00\\00 \\00\\00\\00\"\\00\\00\\00È\\00\\00\\00\\1A\\00\\00\\00\\1B\\00\\00\\00\\1D\\00\\00\\00+\\00\\00\\00Ë\\00\\00\\00É\\00\\00\\00Q\\00\\00\\00V\"\nSearchWin = 3.000000\nMinH = 1.000000\nMinW = 4\n\n[Version Info]\nVersion Number = \"1.0\"", error in=w36) -> (refnum out=w32:refnum<file>, error out=w34:errorcluster)  [unwired: 1 in, 1 out]
      n20 = Close File(refnum=w32, error in=w34) -> (path=w31:path, error out=w33:errorcluster)
    }
    frame True {
      # "We got a file, cpy it to ProgramData"
      n21 = Strip Path(path=w42) -> (stripped path=w44:path)  [unwired: 1 out]
      n22 = call <vilib>:"Check if File or Folder Exists.vi"("error in (no error)"=w47, "path"=w44) -> ("error out"=w46:errorcluster, "file or folder exists?"=w45:bool, "dup path"=w43:path)  [unwired: 7 in]
      n23 = case shown="False" w45 {
        tunnel: [w54 w55] -> w48
        tunnel: w46 -> [w53 w55]
        tunnel: w43 -> [w52 _]
        frame False {
          # "folder doesnt exist"
          n24 = Create Folder(path (use dialog)=w52, error in=w53) -> (error out=w54:errorcluster)  [unwired: 1 in, 2 out]
        }
        frame True {
        }
      }
      n25 = Copy(8:w48, 10:w42, 11:w51) -> (0:w50:errorcluster, 3:w49:path)  [unwired: 2 in, 1 out]
    }
  }
  "error out" <- w10
  "ipf file path" <- w9
